vi "PNS Ausgabefeld einfaerben.vi"(6 "Aktionen":T1=enum."initialisieren", 7 "FeldTyp (Eingang)":refnum<vi>, 11 "PNS Istwerte":refnum<vi>) -> ()   [LabVIEW 2020, in "PNS.lvlib"]
uses:
  PNS.lvlib
  PNS Anlagenuebersicht einfaerben Aktionen.ctl
  Aktionen FGV Grenzwerte.ctl
  Allgemein/allgemeine Sub-VIs.lvlib
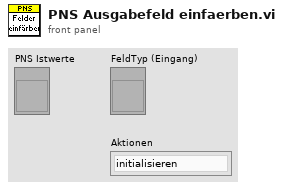
[diagram p1: front panel]
types:
  T1 = typedef "PNS.lvlib/PNS Anlagenuebersicht einfaerben Aktionen.ctl" = enum16{"lesen", "prüfen", "initialisieren"}
  T2 = typedef "PNS.lvlib/Aktionen FGV Grenzwerte.ctl" = enum16{"lesen", "Grenzw. schreiben", "Anweisungscode", "IP-Adresse", "laden", "speichern", "Anweisungscode vorgeben"}
  T3 = typedef "Steuerung PNS.lvclass/Anlegengrenzwerte PNS.ctl" = cluster{"Filter:":T4, "Ventilplatte:":T4, "Heizleitung 1:":T4, "Heizleitung 2:":T4, "Heizleitung 3:":T4, "Heizleitung 4:":T4, "Heizleitung 5:":T4, "Heizleitung 6:":T4}
  T4 = typedef "Steuerung PNS.lvclass/Anlagengrenzwerte Parameteranzeige.ctl" = cluster{"Sollwert":T5, "Warn-Min":T5, "Warn-Max":T5, "Abschalt-Min":T5, "Abschalt-Max":T5, "Regler":u16, "AnlagenParameter":string}
  T5 = typedef "Zahlen-Eingabefeld.ctl" = sgl
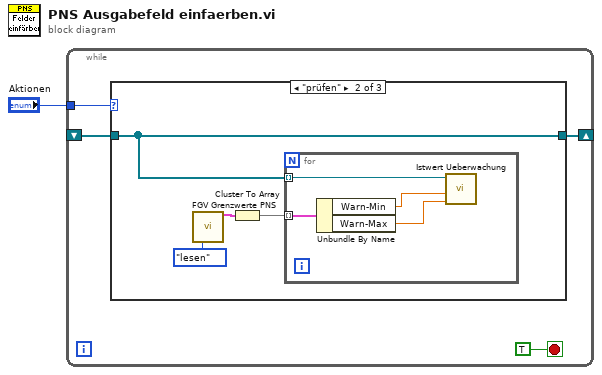
[diagram p0: block diagram]
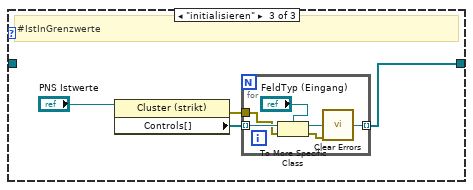
[diagram p3: hidden frame]
diagram:
  n1 = while {
    tunnel: "Aktionen" -> [w4]
    shift-right: [w3] -> _
    shift-left: _ -> [w2]
    stop <- TRUE stop-if-true
    n2 = case shown="\"prüfen\"" w4 {
      tunnel: [w6 w7 w15] -> w3
      tunnel: w2 -> [w6 w7 _]
      frame "lesen", Default {
      }
      frame "prüfen" {
        n3 = call "FGV Grenzwerte PNS.vi"("Aktionen FGV Grenzwerte"=Aktionen_FGV_Grenzwerte."lesen") -> ("Grenzwerte PNS 2"=w9:T3)  [unwired: 12 in, 2 out]
        n4 = Cluster To Array(cluster=w9) -> (array=w8:T4[])
        n5 = for {
          tunnel: w8 -> [w14] mode=indexing
          tunnel: w7 -> [w11] mode=indexing
          n6 = Unbundle By Name(w14) -> ("Warn-Min"=w13:T5, "Warn-Max"=w12:T5)
          n7 = call "Istwert Ueberwachung.vi"("Max"=w12, "Min"=w13, "Referernz"=w11) -> ()  [unwired: 9 in]
        }
      }
      frame "initialisieren" {
        # "#IstInGrenzwerte"
        n8 = property class="Cluster (strikt)"(reference="PNS Istwerte") -> (error out=w16:errorcluster, "Controls[]"=w17:refnum<vi>[])  [unwired: 1 in, 1 out]
        n9 = for {
          tunnel: w17 -> [w23] mode=indexing
          tunnel: [w22] -> w15 mode=indexing
          tunnel: w16 -> [w20]
          n10 = To More Specific Class(target class="FeldTyp (Eingang)", reference=w23, error in=w20) -> (specific class reference=w22:refnum<vi>, error out=w19:errorcluster)
          n11 = call <vilib>:"Clear Errors.vi"("error in (no error)"=w19) -> ()  [unwired: 5 in, 2 out]
        }
      }
    }
  }
